vi "GetVert.vi"(4 "error in":errorcluster, 5 "Card Type":enum16{"DP 110", "DP 310"}(ring), 6 "Channel (1)":i32=1, 7 "InstrumentID":u32) -> (0 "error out":errorcluster, 1 "index of element":i32, 2 "V scale":T2 {"Coupling" items=["DC 1 MOhm", "AC 1 MOhm", "DC 50 Ohm", "AC 50 OHM"]; "Offset" format="%.2f"}, 3 "Instrument ID out":u32)   [LabVIEW 2022 SP3]
uses:
  <instrlib>/Acqiris Dx/Acqiris Dx.lvlib
panel:
  out "Bandwidth":T1(ring)=enum."BWL 200 MHz"
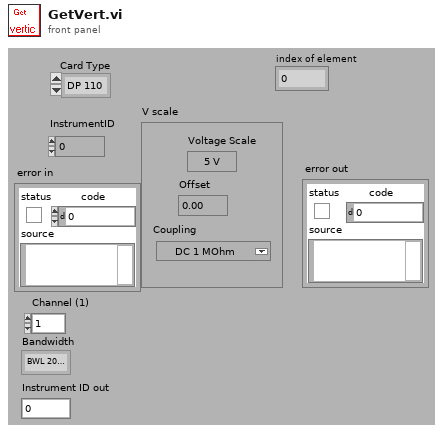
[diagram p1: front panel]
types:
  T1 = enum32{"no bandwidth limit", "BWL 25 MHz", "BWL 700 MHz", "BWL 200 MHz", "BWL 20 MHz", "BWL 35 MHz"}
  T2 = cluster{"Voltage Scale":i16, "Offset":dbl, "Coupling":u16}
  T3 = enum32{"unused", "DC, 1 MOhm", "AC, 1 MOhm", "DC, 50 Ohm", "AC 50 Ohm"}
  T4 = cluster{"index of element":i32, "Offset":dbl, enum32{"unused", "DC, 1 MOhm", "AC, 1 MOhm", "DC, 50 Ohm", "AC 50 Ohm"}}
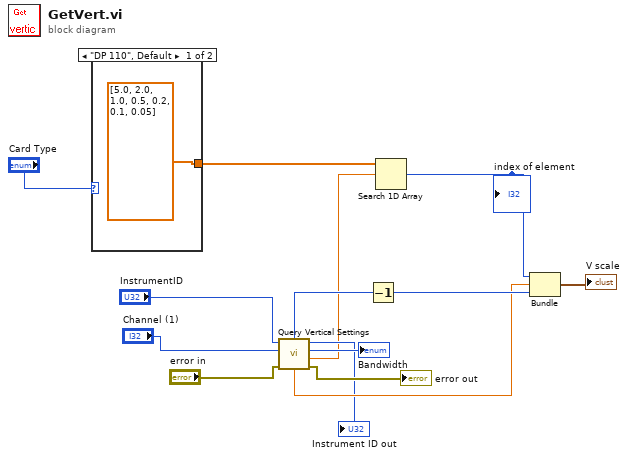
[diagram p0: block diagram]
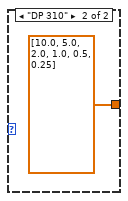
[diagram p2: hidden frame]
diagram:
  n1 = case shown="\"DP 110\", Default" "Card Type" {
    tunnel: [dbl[] [5.0, 2.0, 1.0, 0.5, 0.2, 0.1, 0.05] dbl[] [10.0, 5.0, 2.0, 1.0, 0.5, 0.25]] -> w4
    frame "DP 110", Default {
    }
    frame "DP 310" {
    }
  }
  n2 = call <instrlib>:"Query Vertical Settings.vi"("Instrument ID"="InstrumentID", "Channel (1)"="Channel (1)", "error in (no error)"="error in") -> ("dup Instrument ID"=→"Instrument ID out":u32, "Bandwidth"=→"Bandwidth":T1, "Coupling"=w8:T3, "Full Scale"=w3:dbl, "error out"=→"error out":errorcluster, "Offset"=w6:dbl)  [unwired: 1 out]
  n3 = Decrement(x=w8) -> (x-1=w7:T3)
  n4 = Search 1D Array(1D array=w4, element=w3) -> (index of element=w2:i32)  [unwired: 1 out]
  "index of element" <- w2
  n5 = Bundle("index of element"=w2, "Offset"=w6, w7) -> (→"V scale":T4)  [unwired: 1 out]
